vi "Method 3.vi"(10 "My Input":dbl, 11 "Test Actor 2 in":refnum<class "Test Actor 2.lvclass">) -> (2 "My Output":dbl, 3 "Test Actor 2 out":refnum<class "Test Actor 2.lvclass">)   [LabVIEW 2023, in "Test Actor 2.lvlib" / "Test Actor 2.lvclass"]
doc: "My Method Description"
uses:
  Test Actor 2.lvclass
  Test Actor 2.lvclass/Test Actor 2.ctl
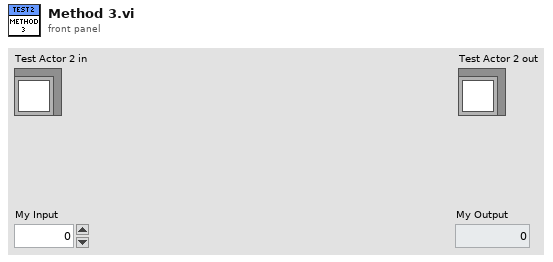
[diagram p1: front panel]
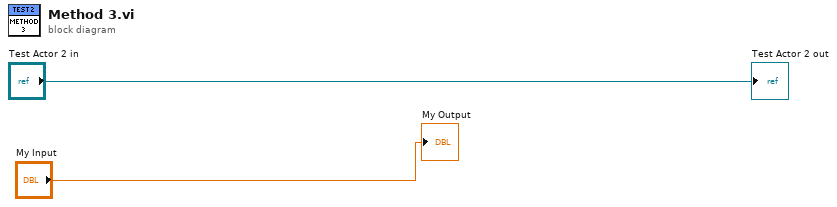
[diagram p0: block diagram]
diagram:
  "Test Actor 2 out" <- "Test Actor 2 in"
  "My Output" <- "My Input"
